vi "lightBarriers.vi"() -> ()   [LabVIEW 2011]
uses:
  C:/Program Files (x86)/National Instruments/LabVIEW 2011/vi.lib/ULx/ULx_LV.dll
  Program Files (x86)/National Instruments/LabVIEW 2011/vi.lib/ULx/ULx_LV.dll
  GlobalDAQ.vi
  <vilib>/ULx/Read.llb/ULx Read (Analog 1D DBL NChan 1Samp).vi
  GlobalSerial.vi
  setPositionServo.vi
  stopDAQ.vi
  stopServos.vi
panel:
  out "program status":T1(ring)
  in  "system info":enum32{"light barriers", "servo motors"}(tab)
  out "light barriers debug output":T2
  out "detection":bool[](array[boolean])
  out "light barrier voltage (V)":dbl[](array[knob]) scale=0.0..15.0
  in  "voltage ref":dbl[](array[slide]) min=0.0 max=10.0 scale=0.0..10.0
  out "servo debug output":T3={"VISA resource name out"="COM3", "error out"={"status"=FALSE, "code"=0, "source"=""}}
  out "serial status":u32(colorbox)
  in  "USB COM port":refnum<visa-resource-name>="COM3"
  out "Stop Reading":bool
  out "fly detected":bool
  in  "stop":bool
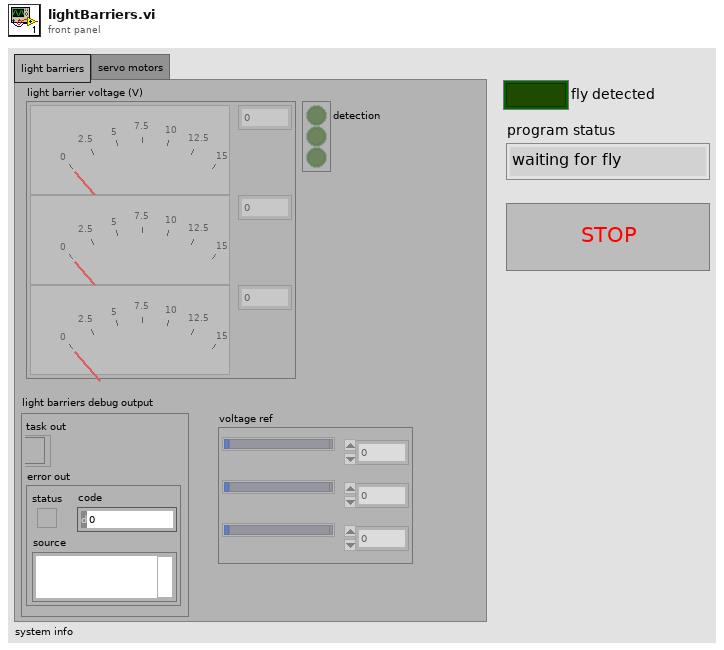
[diagram p1: front panel]
types:
  T1 = enum16{"waiting for fly", "getting ready to blow", "blowing the fly"}
  T2 = cluster{"task out":refnum<k24>, "error out":errorcluster}
  T3 = cluster{"VISA resource name out":refnum<visa-resource-name>, "error out":errorcluster}
  T4 = cluster{"det 0":bool, "det time 0":u32, "det 1":bool, "det time 1":u32, "detected":bool, "detection time":u32}
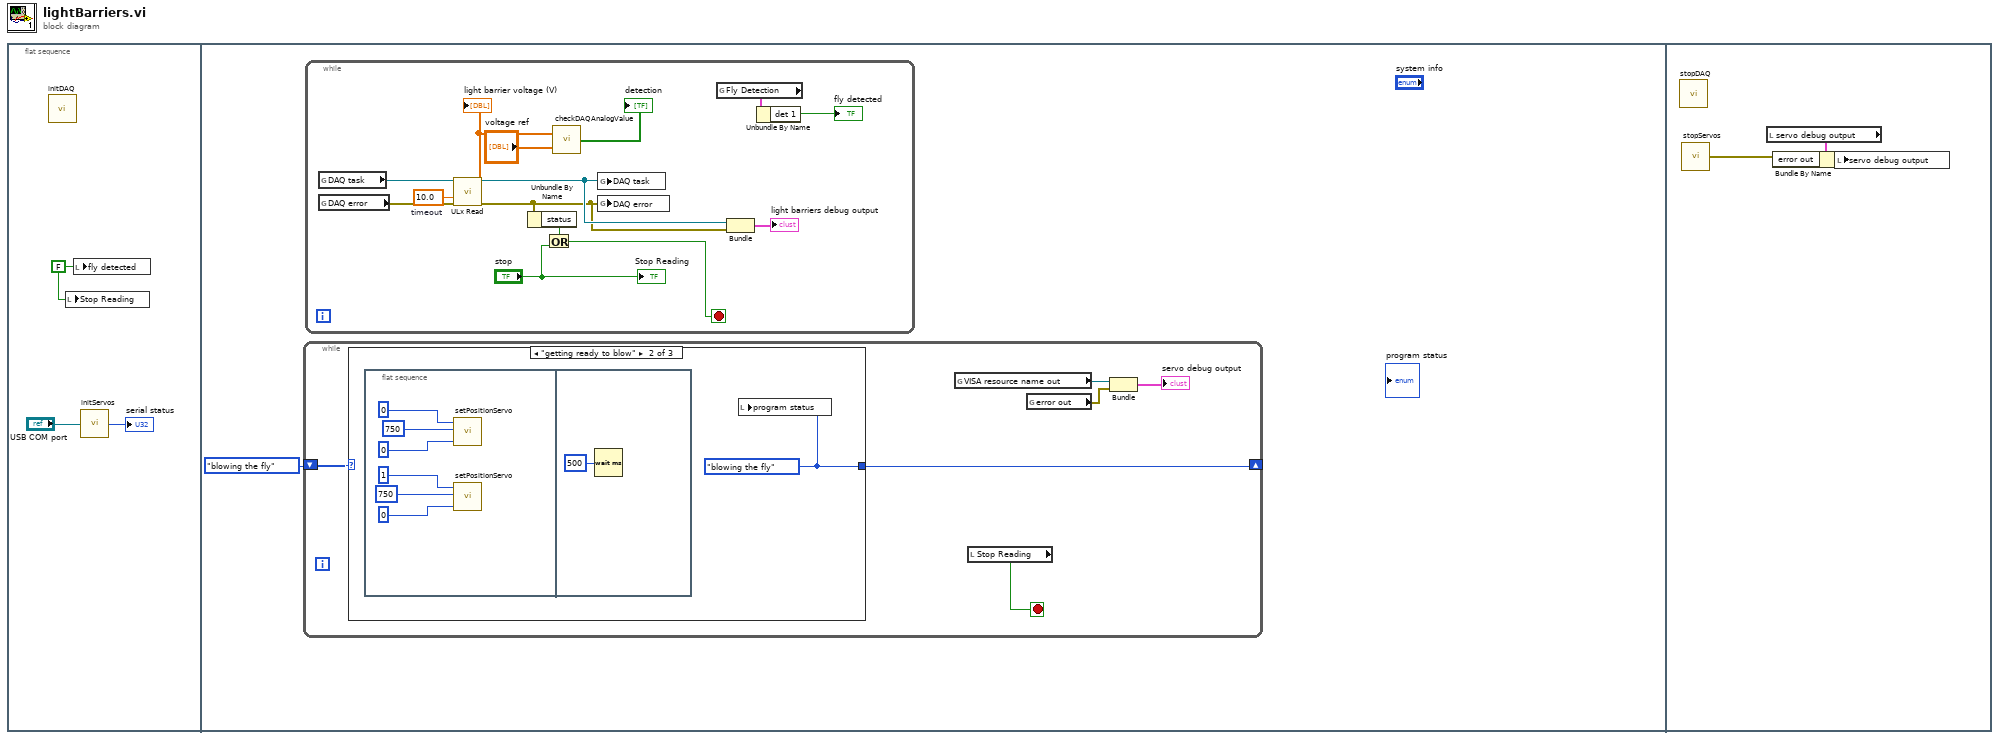
[diagram p0: block diagram]
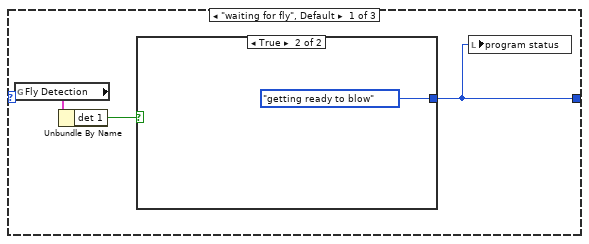
[diagram p2: hidden frame]
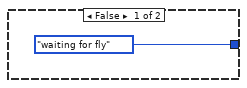
[diagram p3: hidden frame]
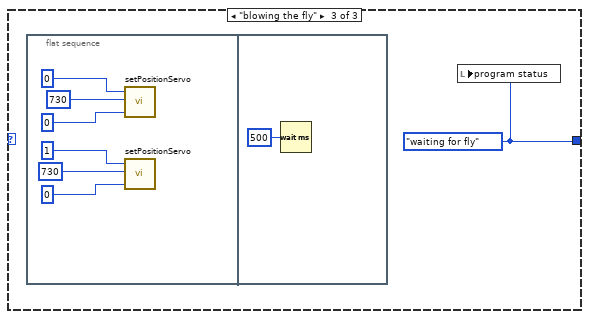
[diagram p4: hidden frame]
diagram:
  n1 = flat-sequence {
    frame #0 {
      w3 = FALSE ("fly detected")
      n2 = call "initDAQ.vi"() -> ()  [unwired: 12 in]
      n3 = local write "Stop Reading"(w3) -> ()
      n4 = local write "fly detected"(w3) -> ()
      n5 = call "initServos.vi"("VISA resource name"="USB COM port") -> ("serial status"=→"serial status":u32)
    }
    frame #1 {
      n6 = while {
        shift-right: [w5] -> _
        shift-left: T1."blowing the fly" -> [w6]
        stop <- w10 stop-if-true
        n7 = case shown="\"getting ready to blow\"" w6 {
          tunnel: [w13 w16 w24] -> w5
          frame "waiting for fly", Default {
            n8 = global read "GlobalDAQ.vi" "Fly Detection"() -> (w12:T4)
            n9 = Unbundle By Name(w12) -> ("det 1"=w11:bool)
            n10 = case shown="True" w11 {
              tunnel: [T1."waiting for fly" T1."getting ready to blow"] -> w13
              frame False {
              }
              frame True {
              }
            }
            n11 = local write "program status"(w13) -> ()
          }
          frame "getting ready to blow" {
            w16 = T1."blowing the fly"
            n12 = flat-sequence {
              frame #0 {
                n13 = call "setPositionServo"("speed"=u8 0, "servo position"=u16 750, "channel"=u8 0) -> ()
                n14 = call "setPositionServo"("speed"=u8 0, "servo position"=u16 750, "channel"=u8 1) -> ()
              }
              frame #1 {
                n15 = Wait (ms)(milliseconds to wait=u32 500) -> ()  [unwired: 1 out]
              }
            }
            n16 = local write "program status"(w16) -> ()
          }
          frame "blowing the fly" {
            w24 = T1."waiting for fly"
            n17 = flat-sequence {
              frame #0 {
                n18 = call "setPositionServo"("speed"=u8 0, "servo position"=u16 730, "channel"=u8 0) -> ()
                n19 = call "setPositionServo"("speed"=u8 0, "servo position"=u16 730, "channel"=u8 1) -> ()
              }
              frame #1 {
                n20 = Wait (ms)(milliseconds to wait=u32 500) -> ()  [unwired: 1 out]
              }
            }
            n21 = local write "program status"(w24) -> ()
          }
        }
        n22 = global read "GlobalSerial.vi" "VISA resource name out"() -> (w9:refnum<visa-resource-name>)
        n23 = local read "Stop Reading"() -> (w10:bool)
        n24 = global read "GlobalSerial.vi" "error out"() -> (w8:errorcluster)
        n25 = Bundle("VISA resource name out"=w9, "error out"=w8) -> (→"servo debug output":T3)  [unwired: 1 in]
      }
      n26 = while {
        stop <- w43 stop-if-true
        w44 = 10.0  # timeout
        n27 = global read "GlobalDAQ.vi" "DAQ task"() -> (w40:refnum<k24>)
        n28 = global read "GlobalDAQ.vi" "DAQ error"() -> (w39:errorcluster)
        n29 = call-poly <vilib>:"ULx Read.vi"("task in"=w40, "timeout"=w44, "error in"=w39) -> ("task out"=w37:refnum<k24>, "data"=w38:dbl[], "error out"=w36:errorcluster)  [unwired: 10 in]
        "light barrier voltage (V)" <- w38
        n30 = Unbundle By Name(w36) -> ("status"=w45:bool)
        n31 = Or(x=w45, y="stop") -> (x .or. y?=w43:bool)
        n32 = call "checkDAQAnalogValue.vi"("Reference"="voltage ref", "Array"=w38) -> ("thresholded analog inputs"=→"detection":bool[])
        n33 = global write "GlobalDAQ.vi" "DAQ task"(w37) -> ()
        n34 = global write "GlobalDAQ.vi" "DAQ error"(w36) -> ()
        n35 = global read "GlobalDAQ.vi" "Fly Detection"() -> (w34:T4)
        n36 = Bundle("task out"=w37, "error out"=w36) -> (→"light barriers debug output":T2)  [unwired: 1 in]
        n37 = Unbundle By Name(w34) -> ("det 1"=→"fly detected":bool)
        "Stop Reading" <- "stop"
      }
    }
    frame #2 {
      n38 = call "stopDAQ"() -> ()  [unwired: 12 in]
      n39 = call "stopServos"() -> ("error out"=w46:errorcluster)  [unwired: 2 in]
      n40 = local read "servo debug output"() -> (w47:T3)
      n41 = Bundle By Name(cluster=w47, "error out"=w46) -> (w48:T3)
      n42 = local write "servo debug output"(w48) -> ()
    }
  }
